vi "Setup.vi"(10 "Actor":refnum<class "Actor.lvclass">, 11 "jettl Queue Actor in":refnum<class "jettl Queue Actor.lvclass">) -> (3 "jettl Queue Actor out":refnum<class "jettl Queue Actor.lvclass">)   [LabVIEW 2021, in "jettl.lvlib" / "jettl Queue Actor.lvlib" / "jettl Queue Actor.lvclass"]
uses:
  jettl Queue Actor.lvclass
  Actor/Actor/Actor.lvclass
  jettl.lvlib
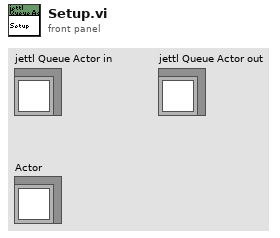
[diagram p1: front panel]
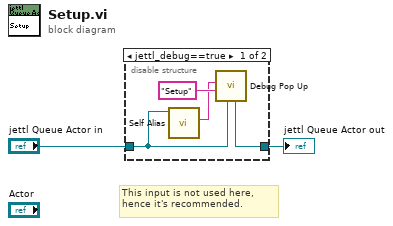
[diagram p0: block diagram]
diagram:
  # "This input is not used here, hence it's recommended."
  n1 = disable-structure shown="jettl_debug==true" {
    disable-tunnel: "jettl Queue Actor in" -> [w3 _]
    disable-tunnel: [w4 _] -> w1
    frame condition #0 (active) {
      n2 = call-dynamic "Self Alias.vi"("jettl Queue Actor in"=w3) -> ("Self Alias"=w5:string)  [unwired: 10 in]
      n3 = call "Debug Pop Up.vi"("Input"=w3, "Method"="Setup", "Alias"=w5) -> ("Output"=w4:refnum<class "jettl Queue Actor.lvclass">)  [unwired: 8 in]
    }
    frame condition #1 {
    }
  }
  "jettl Queue Actor out" <- w1
